vi "tower Controller.vi"(8 "error in":errorcluster) -> ()   [LabVIEW 2017]
doc: "This VI executes continuously carrying out the current operation and responding to updates or new operations. It will often contain the timing or control code that is difficult to place directly in TeleOp. This VI generally opens all sensors and motors and isolates the rest of the robot code from knowing how the operations are carried out."
uses:
  <vilib>/Rock Robotics/WPI/Framework/Completion Status.ctl
  tower Setpoints.ctl
  tower Operations.ctl
  <vilib>/Rock Robotics/SystemInterfaces/DIO/FPGA_DIOChannel.ctl
  <vilib>/Rock Robotics/WPI/Encoder/WPI_EncoderType.ctl
  <vilib>/Rock Robotics/SystemInterfaces/DIO/FPGA_DIOPWMChannel.ctl
  Phoenix-LabVIEW/Motor Controller/Controls/CTRE_Phoenix_MotorControl_ControlMode.ctl
  tower Published Globals.vi
  <vilib>/Rock Robotics/WPI/Counter/WPI_CounterDigitalInputToDigitalSource.vi
  Framework/Robot Global Data.vi
  <vilib>/Rock Robotics/WPI/PWM/WPI_PWMDeviceRef.ctl
  <vilib>/Rock Robotics/WPI/DigitalInput/WPI_DigitalInputDevRef.ctl
  <vilib>/Rock Robotics/SystemInterfaces/Encoder/FPGA_EncoderIdx.ctl
  <vilib>/Rock Robotics/SystemInterfaces/Counter/FPGA_CounterCtrSystemIndex.ctl
  <vilib>/Rock Robotics/WPI/Encoder/WPI_EncoderDevRef.ctl
  <vilib>/Rock Robotics/WPI/MotorControl/WPI_MotorControlType.ctl
  <vilib>/Rock Robotics/WPI/PWM/WPI_PWMDeadband.ctl
  <vilib>/Rock Robotics/WPI/MotorControl/WPI_MotorControlDeviceRef.ctl
  <vilib>/Rock Robotics/Network Tables/NT Write Boolean.vi
panel:
  out "Arm Encoder":dbl
  out "TowerLastCommandStatus":T1=enum."Incomplete"
  in  "Interactive Values":T2
  out "Current\nCmd":string
  in  "Buttons":cluster{"Execute Cmd":bool, "Abort Cmd":bool}
  out "Command Timing":cluster{"Start Time (ms)":u32, "Iterations":i32}
  out "Status":T1
  # "Tip: It may be helpful to observe inputs and sensor values.\nYou may also want to display tuning or debugging controls.\nFor ArmPosition Setpoint is # of raw units to travel\nFor ArmReset Setpoint is motor speed (-1 to +1)\nDuration is #seconds to run (zero is reset is immediate).\n-Motor speed sp lowers arm, + motor speed sp raises arm.\nFor reset, motor will stop when limit swtich is made."
  # "Interactive Command: You may fill in the settings for a command\nand schedule it with the Execute button. You can observe and abort\nany command while fine tuning the code for the controller."
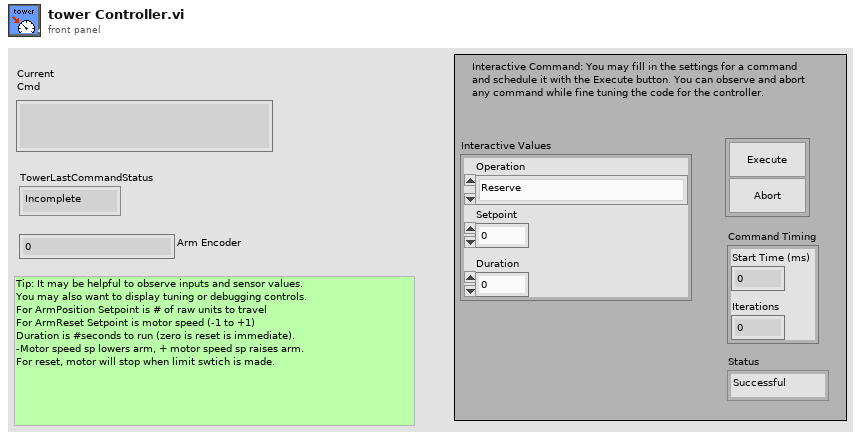
[diagram p1: front panel]
types:
  T1 = typedef "Completion Status.ctl" = enum16{"Successful", "Aborted", "Incomplete"}
  T2 = typedef "tower Setpoints.ctl" = cluster{"Operation":T3, "Setpoint":dbl, "Duration":dbl}
  T3 = typedef "tower Operations.ctl" = enum16{"Reserve", "Read Current", "Immediate", "LaunchClimber", "ArmReset", "ArmPosition", "TowerClimbImmediate", "ArmSpitPosition"}
  T4 = typedef "FPGA_DIOPWMChannel.ctl" = enum8{"PWM 0", "PWM 1", "PWM 2", "PWM 3", "PWM 4", "PWM 5", "PWM 6", "PWM 7", "PWM 8", "PWM 9", "PWM MXP 0", "PWM MXP 1", "PWM MXP 2", "PWM MXP 3", "PWM MXP 4", "PWM MXP 5", "PWM MXP 6", "PWM MXP 7", "PWM MXP 8", "PWM MXP 9", "Invalid"}
  T5 = typedef "WPI_EncoderType.ctl" = enum16{"1x", "2x", "4x"}
  T6 = typedef "FPGA_DIOChannel.ctl" = enum8{"DIO 0", "DIO 1", "DIO 2", "DIO 3", "DIO 4", "DIO 5", "DIO 6", "DIO 7", "DIO 8", "DIO 9", "DIO MXP 0", "DIO MXP 1", "DIO MXP 2", "DIO MXP 3", "DIO MXP 4", "DIO MXP 5", "DIO MXP 6", "DIO MXP 7", "DIO MXP 8", "DIO MXP 9", "DIO MXP 10", "DIO MXP 11", "DIO MXP 12", "DIO MXP 13", "DIO MXP 14", "DIO MXP 15", "SPI Port CS1", "SPI Port CS2", "SPI Port CS3", "SPI Port MISO", "SPI Port MOSI", "Invalid"}
  T7 = typedef "WPI_PWMDeviceRef.ctl" = cluster{"DeviceStatus":errorcluster, "PWM Channel":T4}
  T8 = typedef "WPI_EncoderDevRef.ctl" = cluster{"DevStatus":errorcluster, "EncoderIndex":T9, "CounterIndex":T10, "DistancePerCount":dbl, "Decoding Type":T5}
  T9 = typedef "FPGA_EncoderIdx.ctl" = enum8{"Enc 0", "Enc 1", "Enc 2", "Enc 3", "Enc 4", "Enc 5", "Enc 6", "Enc 7", "Invalid"}
  T10 = typedef "FPGA_CounterCtrSystemIndex.ctl" = enum8{"Ctr 0", "Ctr 1", "Ctr 2", "Ctr 3", "Ctr 4", "Ctr 5", "Ctr 6", "Ctr 7", "Invalid"}
  T11 = typedef "WPI_DigitalInputDevRef.ctl" = cluster{"DevStatus":errorcluster, "DIO Channel":T6}
  T12 = typedef "WPI_DigitalOutputDevRef.ctl" = cluster{"DIO Channel":T6, "DevStatus":errorcluster}
  T13 = typedef "FPGA_CounterEncoderSourceConvertionLVSourceType.ctl" = cluster{"DevStatus":errorcluster, "AnalogTriggerMode?":bool, "DigitalMode":cluster{"DIO Channel":T14}, "AnalogTriggerMode":cluster{"AnalogTriggerIndex":T15, "OutputType":T16}}
  T14 = typedef "FPGA_DIODigitalSourceChannel.ctl" = enum8{"DIO 0", "DIO 1", "DIO 2", "DIO 3", "DIO 4", "DIO 5", "DIO 6", "DIO 7", "DIO 8", "DIO 9", "DIO MXP 0", "DIO MXP 1", "DIO MXP 2", "DIO MXP 3", "DIO MXP 4", "DIO MXP 5", "DIO MXP 6", "DIO MXP 7", "DIO MXP 8", "DIO MXP 9", "DIO MXP 10", "DIO MXP 11", "DIO MXP 12", "DIO MXP 13", "DIO MXP 14", "DIO MXP 15", "Disabled"}
  T15 = typedef "FPGA_AnalogTriggerIndex.ctl" = enum8{"Trig 0", "Trig 1", "Trig 2", "Trig 3", "Trig 4", "Trig 5", "Trig 6", "Trig 7", "Invalid"}
  T16 = typedef "FPGA_AnalogTriggerOutType.ctl" = enum16{"InWindow", "TriggerState", "Rising", "Falling"}
  T17 = typedef "WPI_MotorControlDeviceRef.ctl" = cluster{"DeviceStatus":errorcluster, "Type":T18, "PWM":cluster{"PWM Channel":T4, "DeadBand":T19}, "CAN":cluster{"Device Number":u8, "SetOutput VI Ref":variant, "GetOutput VI Ref":variant, "Enable VI Ref":variant, "Disable VI Ref":variant, "Data":variant}, "Invert":bool, "DIO PWM":cluster{"PWM \"Enable\" Channel":T4, "DIOChannel":T6, "PWM Rate":dbl}}
  T18 = typedef "WPI_MotorControlType.ctl" = enum16{"PWM", "CAN", "DIO PWM"}
  T19 = typedef "WPI_PWMDeadband.ctl" = cluster{"Name":string, "maxPositivePwm":i32, "minPositivePwm":i32, "centerPwm":i32, "maxNegativePwm":i32, "minNegativePwm":i32, "angularRange":u16}
  T20 = typedef "Command Status Info.ctl" = cluster{"Name":string, "Status":T1, "notifier out":T21}
  T21 = typedef "Completion Notifier.ctl" = refnum<notifier>
  T22 = cluster{"Current Command":T2, "Command Timing":cluster{"Start Time (ms)":u32, "Iterations":i32}, "Command Arguments":cluster{"Command Info":T20, "Description":string, "Default Command":T2, "queue out":refnum<queue>, "Subsystem Name":string}}
  T23 = typedef "CTRE_Phoenix_MotorControl_ControlMode.ctl" = u16
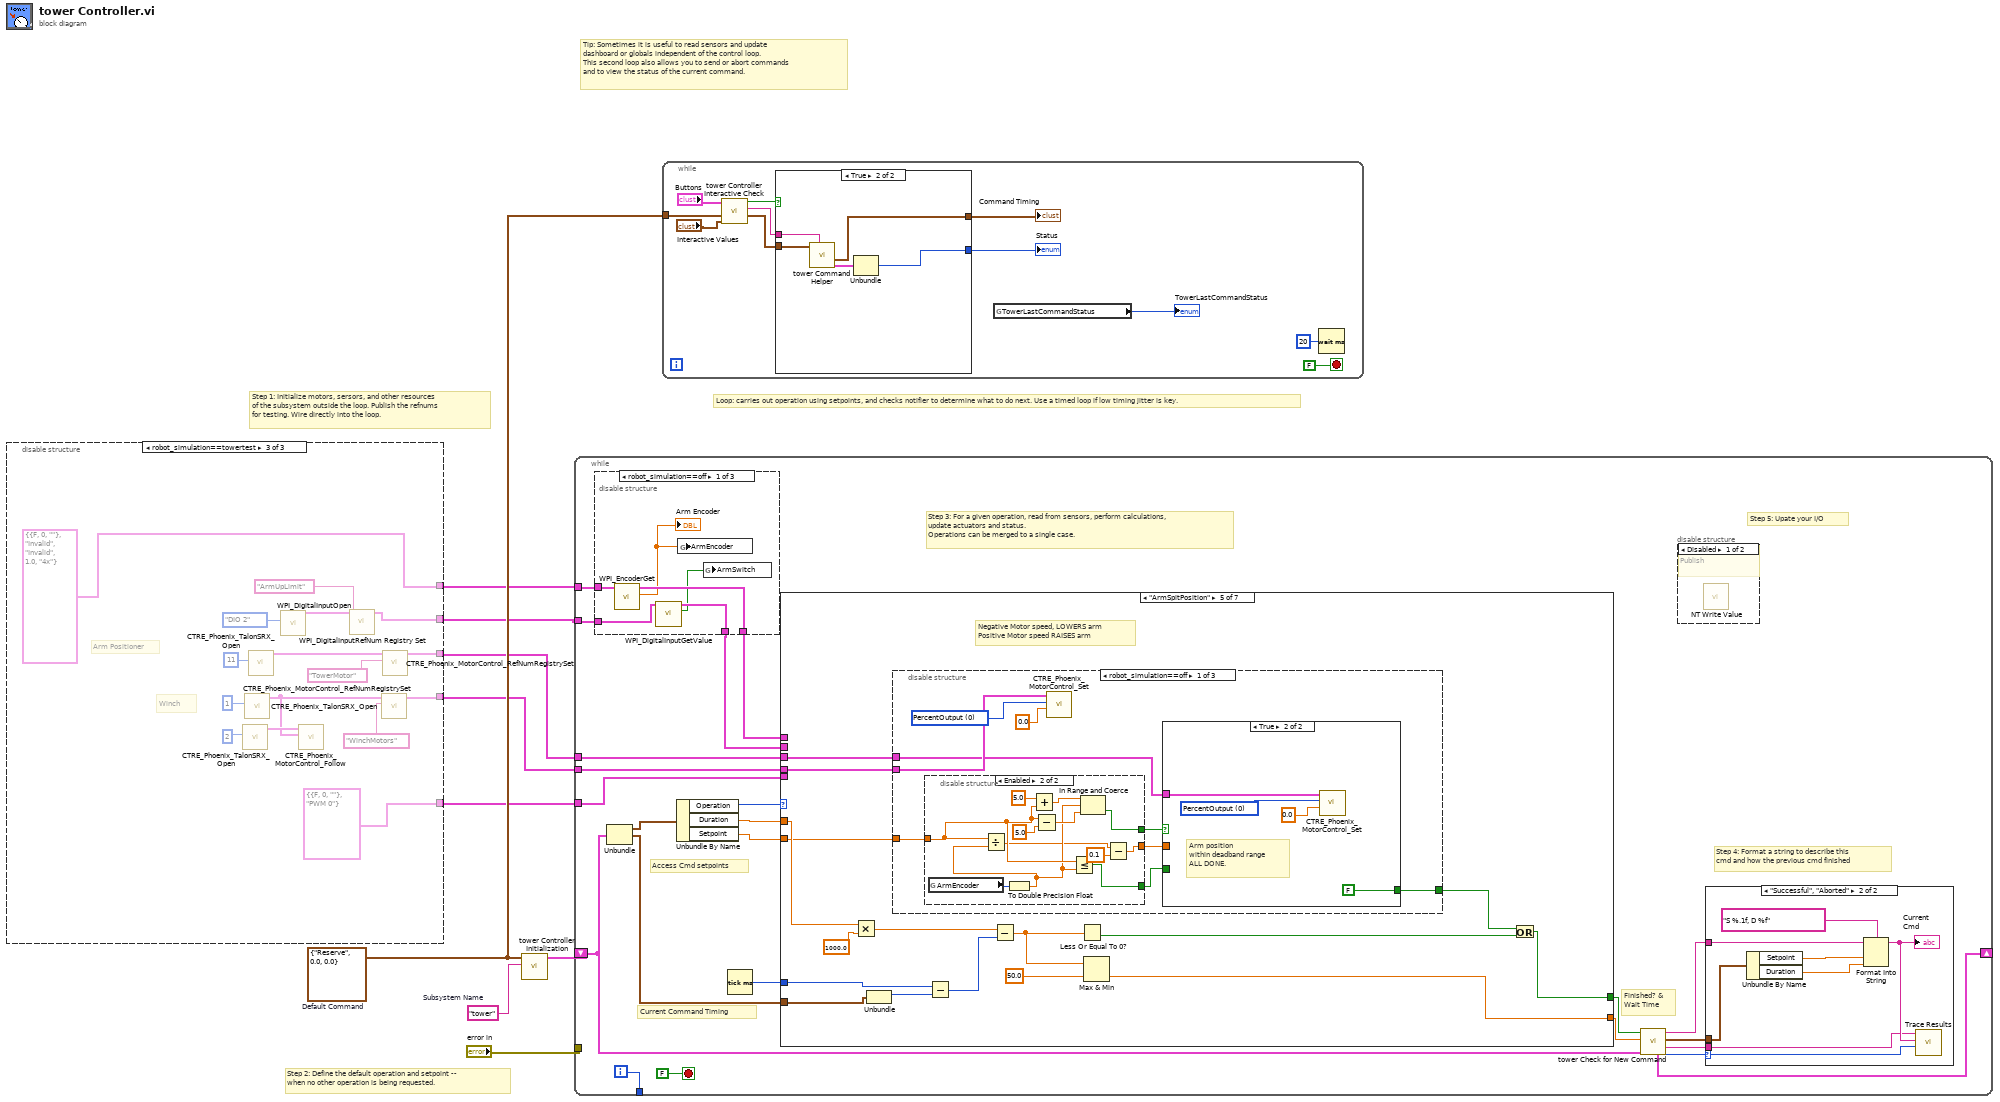
[diagram p0: block diagram]
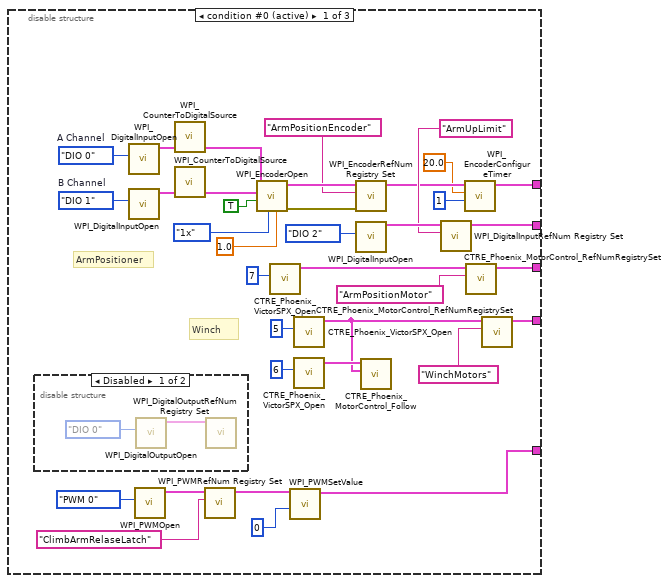
[diagram p2: hidden frame]
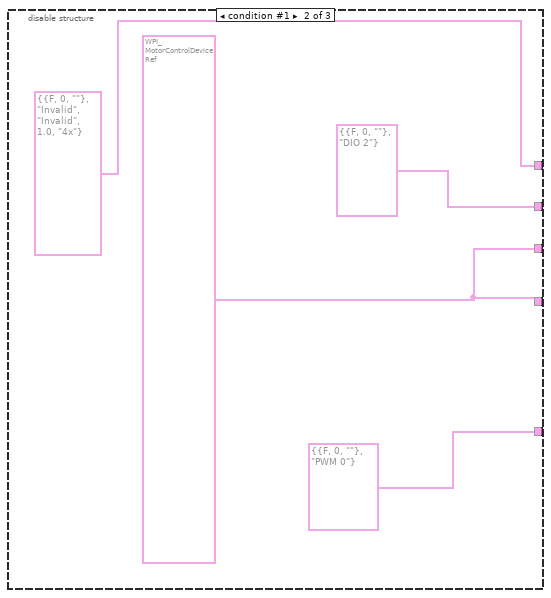
[diagram p4: hidden frame]
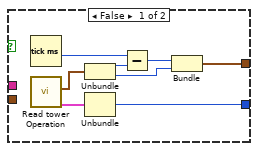
[diagram p5: hidden frame]
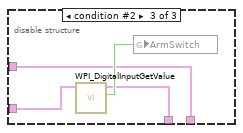
[diagram p7: hidden frame]
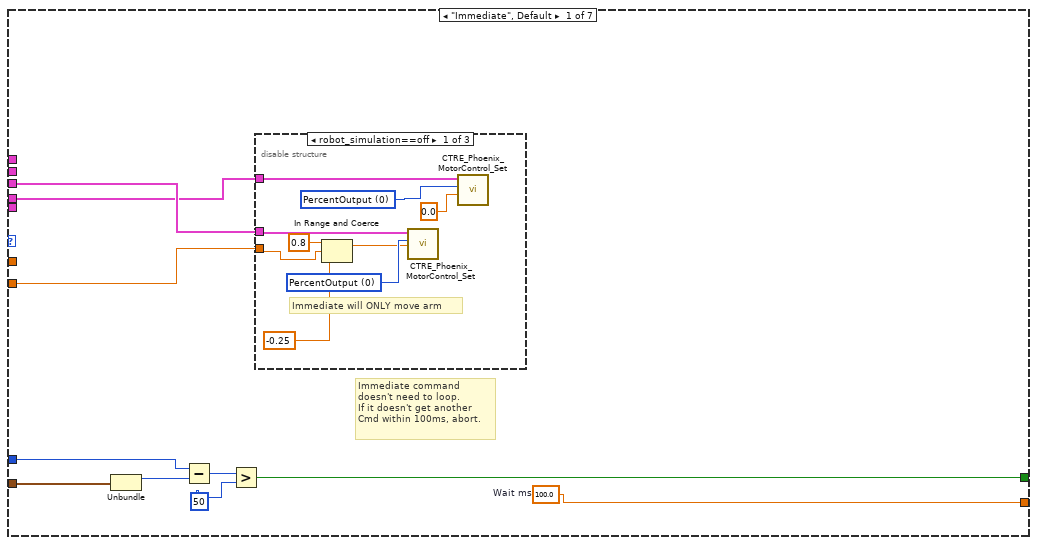
[diagram p10: hidden frame]
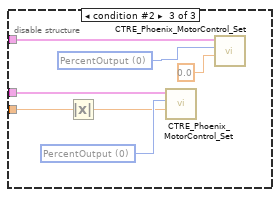
[diagram p12: hidden frame]
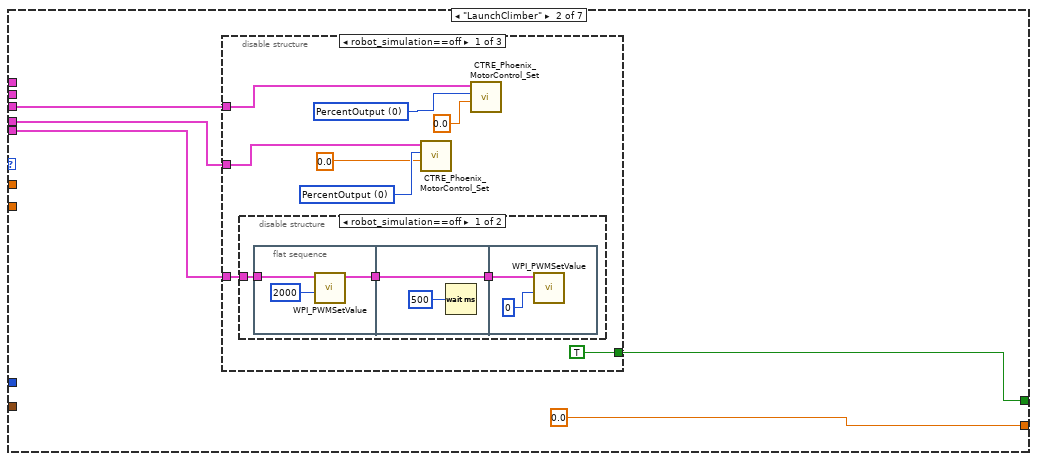
[diagram p13: hidden frame]
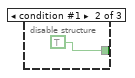
[diagram p15: hidden frame]
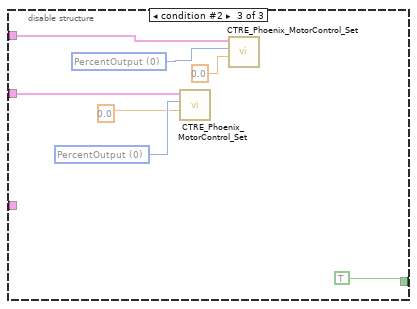
[diagram p16: hidden frame]
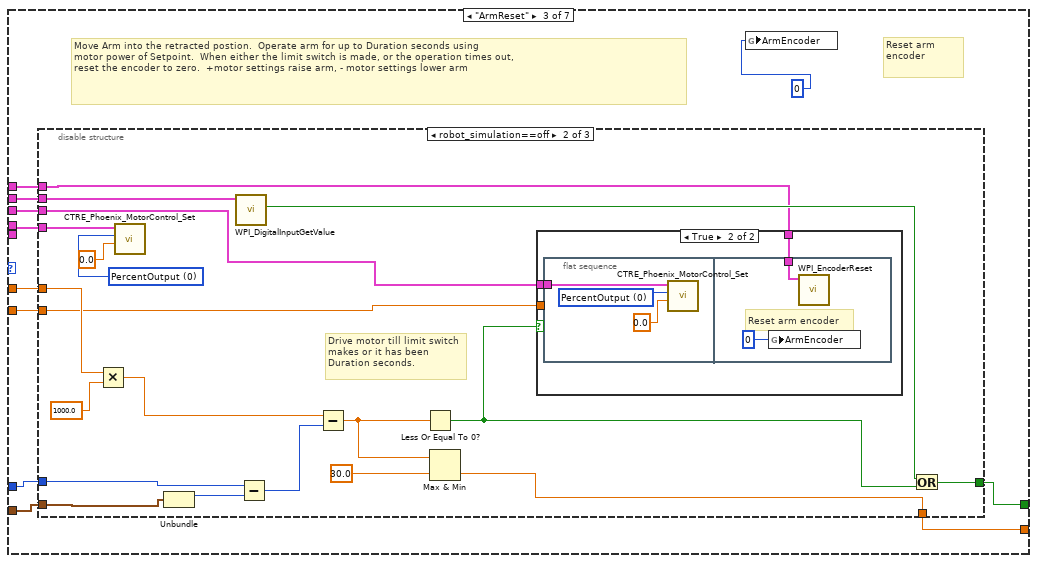
[diagram p17: hidden frame]
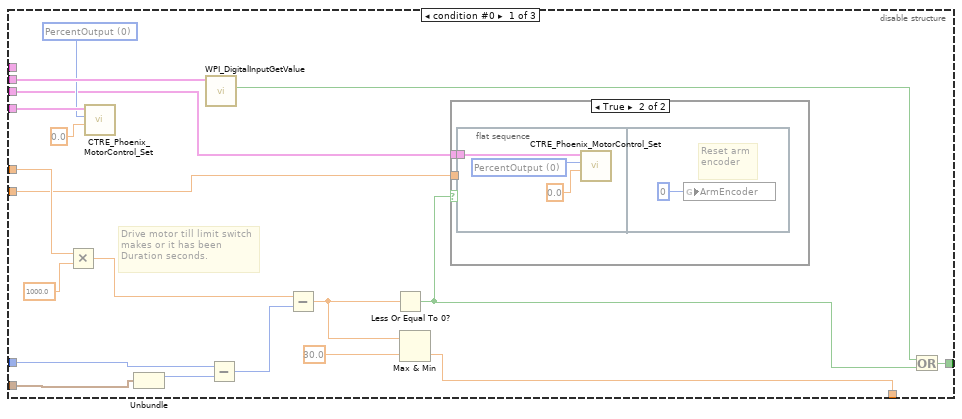
[diagram p18: hidden frame]
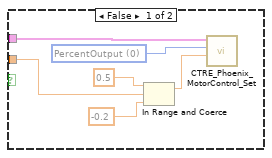
[diagram p19: hidden frame]
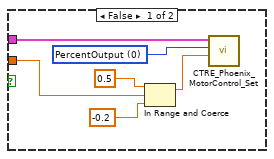
[diagram p20: hidden frame]
diagram:
  w6 = T2 {"Operation"=enum."Reserve", "Setpoint"=0.0, "Duration"=0.0}  # Default Command
  w7 = "tower"  # Subsystem Name
  # "Tip: Sometimes it is useful to read sensors and update\ndashboard or globals independent of the control loop.\nThis second loop also allows you to send or abort commands\nand to view the status of the current command."
  # "Step 2: Define the default operation and setpoint --\nwhen no other operation is being requested."
  # "Step 1: Initialize motors, sersors, and other resources\nof the subsystem outside the loop. Publish the refnums\nfor testing. Wire directly into the loop."
  # "Loop: carries out operation using setpoints, and checks notifier to determine what to do next. Use a timed loop if low timing jitter is key."
  n1 = disable-structure shown="robot_simulation==towertest" {
    disable-tunnel: [w37 w48 w65] -> w5
    disable-tunnel: [w40 w48 w61] -> w4
    disable-tunnel: [w22 T8 {"DevStatus"={"status"=FALSE, "code"=0, "source"=""}, "EncoderIndex"=enum."Invalid", "CounterIndex"=enum."Invalid", "DistancePerCount"=1.0, "Decoding Type"=enum."4x"} ("EncoderDevRef") T8 {"DevStatus"={"status"=FALSE, "code"=0, "source"=""}, "EncoderIndex"=enum."Invalid", "CounterIndex"=enum."Invalid", "DistancePerCount"=1.0, "Decoding Type"=enum."4x"} ("EncoderDevRef")] -> w1
    disable-tunnel: [w24 T11 {"DevStatus"={"status"=FALSE, "code"=0, "source"=""}, "DIO Channel"=enum."DIO 2"} ("DigitalInputDevRef") w53] -> w2
    disable-tunnel: [w13 T7 {"DeviceStatus"={"status"=FALSE, "code"=0, "source"=""}, "PWM Channel"=enum."PWM 0"} ("PWMDeviceRef") T7 {"DeviceStatus"={"status"=FALSE, "code"=0, "source"=""}, "PWM Channel"=enum."PWM 0"} ("PWMDeviceRef")] -> w3
    frame condition #0 (active) {
      w35 = FPGA_DIOChannel."DIO 1"  # B Channel
      w34 = FPGA_DIOChannel."DIO 0"  # A Channel
      # "Winch"
      # "ArmPositioner"
      n2 = disable-structure shown="Disabled" {
        frame Disabled {
          n3 = call <vilib>:"WPI_DigitalOutputOpen.vi"("DIO Channel"=FPGA_DIOChannel."DIO 0") -> ("DigitalOutputDevRef"=w47:T12)  [unwired: 9 in, 1 out]
          n4 = call <vilib>:"WPI_DigitalOutputRefNum Registry Set.vi"("DigitalOutputDevRef"=w47) -> ()  [unwired: 9 in, 2 out]
        }
        frame Enabled {
        }
      }
      n5 = call <vilib>:"WPI_DigitalInputOpen.vi"("DIO Channel"=w34) -> ("DigitalInputDevRef"=w31:T11)  [unwired: 1 in, 9 out]
      n6 = call <vilib>:"WPI_DigitalInputOpen.vi"("DIO Channel"=w35) -> ("DigitalInputDevRef"=w32:T11)  [unwired: 1 in, 9 out]
      n7 = call <vilib>:"WPI_PWMOpen.vi"("PWM Channel"=FPGA_DIOPWMChannel."PWM 0") -> ("PWMDeviceRef"=w16:T7)  [unwired: 9 in, 1 out]
      n8 = call-poly <vilib>:"WPI_CounterToDigitalSource.vi"("DigitalInputDevRef"=w31) -> ("Digital Source"=w30:T13)  [unwired: 6 out]
      n9 = call-poly <vilib>:"WPI_CounterToDigitalSource.vi"("DigitalInputDevRef"=w32) -> ("Digital Source"=w33:T13)  [unwired: 6 out]
      n10 = call <vilib>:"WPI_PWMRefNum Registry Set.vi"("refnum name"="ClimbArmRelaseLatch", "PWMDeviceRef"=w16) -> ("PWMDeviceRef"=w15:T7)  [unwired: 8 in, 1 out]
      n11 = call <vilib>:"WPI_EncoderOpen.vi"("DistancePerCount"=1.0, "Decoding Type"=WPI_EncoderType."1x", "Invert Direction (False)"=TRUE, "BSource"=w33, "ASource"=w30) -> ("error out"=w29:errorcluster, "EncoderDevRef"=w28:T8)  [unwired: 3 in, 2 out]
      n12 = call "CTRE_Phoenix_VictorSPX_Open.vi"("Device Number"=u8 7) -> ("CAN Talon SRX Ref"=w38:T17)  [unwired: 9 in, 1 out]
      n13 = call <vilib>:"WPI_PWMSetValue.vi"("Value"=u16 0, "PWMDeviceRef"=w15) -> ("PWMDeviceRef"=w13:T7)  [unwired: 8 in, 1 out]
      n14 = call "CTRE_Phoenix_VictorSPX_Open.vi"("Device Number"=u8 5) -> ("CAN Talon SRX Ref"=w41:T17)  [unwired: 9 in, 1 out]
      n15 = call "CTRE_Phoenix_VictorSPX_Open.vi"("Device Number"=u8 6) -> ("CAN Talon SRX Ref"=w42:T17)  [unwired: 9 in, 1 out]
      n16 = call <vilib>:"WPI_EncoderRefNum Registry Set.vi"("error in (no error)"=w29, "refnum name"="ArmPositionEncoder", "EncoderDevRef"=w28) -> ("EncoderDevRef"=w21:T8)  [unwired: 7 in, 1 out]
      n17 = call <vilib>:"WPI_DigitalInputOpen.vi"("DIO Channel"=FPGA_DIOChannel."DIO 2") -> ("DigitalInputDevRef"=w25:T11)  [unwired: 9 in, 1 out]
      n18 = call "CTRE_Phoenix_MotorControl_Follow.vi"("Master Controller to Follow"=w41, "PhoenixMotorControlDevRef"=w42) -> ()  [unwired: 8 in, 2 out]
      n19 = call <vilib>:"WPI_DigitalInputRefNum Registry Set.vi"("refnum name"="ArmUpLimit", "DigitalInputDevRef"=w25) -> ("DigitalInputDevRef"=w24:T11)  [unwired: 8 in, 1 out]
      n20 = call <vilib>:"WPI_EncoderConfigureTimer.vi"("Number Samples to Average"=u8 1, "Minimum Rate"=20.0, "EncoderDevRef"=w21) -> ("EncoderDevRef"=w22:T8)  [unwired: 7 in, 1 out]
      n21 = call "CTRE_Phoenix_MotorControl_RefNumRegistrySet.vi"("refnum name"="ArmPositionMotor", "PhoenixMotorControlDevRef"=w38) -> ("PhoenixMotorControlDevRef"=w37:T17)  [unwired: 8 in, 1 out]
      n22 = call "CTRE_Phoenix_MotorControl_RefNumRegistrySet.vi"("refnum name"="WinchMotors", "PhoenixMotorControlDevRef"=w41) -> ("PhoenixMotorControlDevRef"=w40:T17)  [unwired: 8 in, 1 out]
    }
    frame condition #1 {
      w48 = T17 {"DeviceStatus"={"status"=FALSE, "code"=0, "source"=""}, "Type"=enum."PWM", "PWM"={"PWM Channel"=enum."Invalid", "DeadBand"={"Name"="", "maxPositivePwm"=0, "minPositivePwm"=0, "centerPwm"=0, "maxNegativePwm"=0, "minNegativePwm"=0, "angularRange"=0}}, "CAN"={"Device Number"=0, "SetOutput VI Ref"=variant, "GetOutput VI Ref"=variant, "Enable VI Ref"=variant, "Disable VI Ref"=variant, "Data"=variant}, "Invert"=FALSE, "DIO PWM"={"PWM \"Enable\" Channel"=enum."Invalid", "DIOChannel"=enum."Invalid", "PWM Rate"=0.0}} ("PhoenixMotorControlDevRef")
    }
    frame condition #2 {
      # "Winch"
      # "Arm Positioner"
      n23 = call "CTRE_Phoenix_TalonSRX_Open.vi"("Device Number"=u8 2) -> ("CAN Talon SRX Ref"=w59:T17)  [unwired: 9 in, 1 out]
      n24 = call "CTRE_Phoenix_TalonSRX_Open.vi"("Device Number"=u8 1) -> ("CAN Talon SRX Ref"=w58:T17)  [unwired: 9 in, 1 out]
      n25 = call "CTRE_Phoenix_TalonSRX_Open.vi"("Device Number"=u8 11) -> ("CAN Talon SRX Ref"=w66:T17)  [unwired: 9 in, 1 out]
      n26 = call <vilib>:"WPI_DigitalInputOpen.vi"("DIO Channel"=FPGA_DIOChannel."DIO 2") -> ("DigitalInputDevRef"=w55:T11)  [unwired: 9 in, 1 out]
      n27 = call "CTRE_Phoenix_MotorControl_Follow.vi"("Master Controller to Follow"=w58, "PhoenixMotorControlDevRef"=w59) -> ()  [unwired: 8 in, 2 out]
      n28 = call <vilib>:"WPI_DigitalInputRefNum Registry Set.vi"("refnum name"="ArmUpLimit", "DigitalInputDevRef"=w55) -> ("DigitalInputDevRef"=w53:T11)  [unwired: 8 in, 1 out]
      n29 = call "CTRE_Phoenix_MotorControl_RefNumRegistrySet.vi"("refnum name"="WinchMotors", "PhoenixMotorControlDevRef"=w58) -> ("PhoenixMotorControlDevRef"=w61:T17)  [unwired: 8 in, 1 out]
      n30 = call "CTRE_Phoenix_MotorControl_RefNumRegistrySet.vi"("refnum name"="TowerMotor", "PhoenixMotorControlDevRef"=w66) -> ("PhoenixMotorControlDevRef"=w65:T17)  [unwired: 8 in, 1 out]
    }
  }
  n31 = call "tower Controller Initialization.vi"("Subsystem Name"=w7, "Default Command"=w6) -> ("Current Command"=w8:T22)  [unwired: 9 in]
  n32 = while {
    shift-right: [w82] -> _
    shift-left: w8 -> [w77]
    tunnel: [w89] -> _
    tunnel: "error in" -> [_]
    tunnel: w5 -> [w76]
    tunnel: w4 -> [w75]
    tunnel: w1 -> [w68]
    tunnel: w2 -> [w72]
    tunnel: w3 -> [w71]
    i -> [w89]
    stop <- FALSE stop-if-true
    # "Step 5: Upate your I/O"
    # "Step 4: Format a string to describe this\ncmd and how the previous cmd finished"
    # "Current Command Timing"
    # "Access Cmd setpoints"
    # "Finished? &\nWait Time"
    # "Step 3: For a given operation, read from sensors, perform calculations,\nupdate actuators and status.\nOperations can be merged to a single case."
    n33 = disable-structure shown="robot_simulation==off" {
      disable-tunnel: w68 -> [w92 w98 w99]
      disable-tunnel: [w96 w98 w99] -> w74
      disable-tunnel: w72 -> [w95 w97 w101]
      disable-tunnel: [w94 w97 w100] -> w73
      frame condition #0 (active) {
        n34 = call <vilib>:"WPI_EncoderGet.vi"("EncoderDevRef"=w92) -> ("Distance"=w91:dbl, "EncoderDevRef"=w96:T8)  [unwired: 5 in, 4 out]
        "Arm Encoder" <- w91
        n35 = call <vilib>:"WPI_DigitalInputGetValue.vi"("DigitalInputDevRef"=w95) -> ("Value"=w93:bool, "DigitalInputDevRef"=w94:T11)  [unwired: 8 in, 1 out]
        n36 = global write "Robot Global Data.vi" "ArmEncoder"(w91) -> ()
        n37 = global write "Robot Global Data.vi" "ArmSwitch"(w93) -> ()
      }
      frame condition #1 {
      }
      frame condition #2 {
        n38 = call <vilib>:"WPI_DigitalInputGetValue.vi"("DigitalInputDevRef"=w101) -> ("Value"=w102:bool, "DigitalInputDevRef"=w100:T11)  [unwired: 8 in, 1 out]
        n39 = global write "Robot Global Data.vi" "ArmSwitch"(w102) -> ()
      }
    }
    n40 = Unbundle(w77) -> ("Current Command"=w88:T2, "Command Timing"=w84:cluster{"Start Time (ms)":u32, "Iterations":i32})  [unwired: 1 out]
    n41 = Unbundle By Name(w88) -> ("Operation"=w87:T3, "Duration"=w86:dbl, "Setpoint"=w83:dbl)
    n42 = Tick Count (ms)() -> (millisecond timer value=w85:u32)
    n43 = case shown="\"ArmSpitPosition\"" w87 {
      tunnel: [w120 0.0 ("Infinite") w169 w253 w301 100.0 w379] -> w69
      tunnel: [w114 w137 w170 w250 w298 FALSE ("ignore previous (F)") w380] -> w70
      tunnel: w84 -> [w116 _ w172 w255 w303 _ w382]
      tunnel: w86 -> [_ _ w174 w252 w300 _ _]
      tunnel: w85 -> [w115 _ w171 w254 w302 _ w381]
      tunnel: w83 -> [w112 _ w173 w247 w295 _ w378]
      tunnel: w76 -> [w113 w139 w177 w246 w294 w363 w376]
      tunnel: w75 -> [w111 w140 w175 w251 w299 w362 w377]
      tunnel: w74 -> [_ _ w176 _ _ _ _]
      tunnel: w73 -> [_ _ w178 _ _ _ _]
      tunnel: w71 -> [_ w138 _ _ _ _ _]
      frame "Immediate", Default {
        w120 = 100.0  # Wait ms
        # "Immediate command\ndoesn't need to loop.\nIf it doesn't get another\nCmd within 100ms, abort."
        n44 = Unbundle(w116) -> ("Start Time (ms)"=w119:u32)  [unwired: 1 out]
        n45 = Subtract(x=w115, y=w119) -> (x-y=w118:u32)
        n46 = Greater?(x=w118, y=u8 50 ("Left Motor")) -> (0:w114:bool)
        n47 = disable-structure shown="robot_simulation==off" {
          disable-tunnel: w113 -> [w129 _ w136]
          disable-tunnel: w112 -> [w122 _ w134]
          disable-tunnel: w111 -> [w125 _ w130]
          frame condition #0 (active) {
            w126 = T23 0 items=["PercentOutput"=0, "Position"=1, "Velocity"=2, "Current"=3, "Follower"=5, "MotionProfile"=6, "MotionMagic"=7, "MotionMagicArc"=8, "MotionProfileArc"=10, "Disabled"=15] ("Control Mode")
            w128 = T23 0 items=["PercentOutput"=0, "Position"=1, "Velocity"=2, "Current"=3, "Follower"=5, "MotionProfile"=6, "MotionMagic"=7, "MotionMagicArc"=8, "MotionProfileArc"=10, "Disabled"=15] ("Control Mode")
            # "Immediate will ONLY move arm"
            n48 = In Range and Coerce(upper limit=0.8, x=w122, lower limit=-0.25) -> (coerced(x)=w121:dbl)  [unwired: 1 out]
            n49 = call "CTRE_Phoenix_MotorControl_Set.vi"("Output"=w121, "Control Mode"=w128, "PhoenixMotorControlDevRef"=w129) -> ()  [unwired: 7 in, 2 out]
            n50 = call "CTRE_Phoenix_MotorControl_Set.vi"("Output"=0.0, "Control Mode"=w126, "PhoenixMotorControlDevRef"=w125) -> ()  [unwired: 7 in, 2 out]
          }
          frame condition #1 {
          }
          frame condition #2 {
            w131 = T23 0 items=["PercentOutput"=0, "Position"=1, "Velocity"=2, "Current"=3, "Follower"=5, "MotionProfile"=6, "MotionMagic"=7, "MotionMagicArc"=8, "MotionProfileArc"=10, "Disabled"=15] ("Control Mode")
            w135 = T23 0 items=["PercentOutput"=0, "Position"=1, "Velocity"=2, "Current"=3, "Follower"=5, "MotionProfile"=6, "MotionMagic"=7, "MotionMagicArc"=8, "MotionProfileArc"=10, "Disabled"=15] ("Control Mode")
            n51 = Absolute Value(x=w134) -> (abs(x)=w133:dbl)
            n52 = call "CTRE_Phoenix_MotorControl_Set.vi"("Output"=w133, "Control Mode"=w135, "PhoenixMotorControlDevRef"=w136) -> ()  [unwired: 7 in, 2 out]
            n53 = call "CTRE_Phoenix_MotorControl_Set.vi"("Output"=0.0, "Control Mode"=w131, "PhoenixMotorControlDevRef"=w130) -> ()  [unwired: 7 in, 2 out]
          }
        }
      }
      frame "LaunchClimber" {
        n54 = disable-structure shown="robot_simulation==off" {
          disable-tunnel: w140 -> [w144 _ w167]
          disable-tunnel: w139 -> [w145 _ w163]
          disable-tunnel: w138 -> [w143 _ _]
          disable-tunnel: [TRUE ("ignore previous (F)") TRUE ("ignore previous (F)") TRUE ("ignore previous (F)")] -> w137
          frame condition #0 (active) {
            w147 = T23 0 items=["PercentOutput"=0, "Position"=1, "Velocity"=2, "Current"=3, "Follower"=5, "MotionProfile"=6, "MotionMagic"=7, "MotionMagicArc"=8, "MotionProfileArc"=10, "Disabled"=15] ("Control Mode")
            w149 = T23 0 items=["PercentOutput"=0, "Position"=1, "Velocity"=2, "Current"=3, "Follower"=5, "MotionProfile"=6, "MotionMagic"=7, "MotionMagicArc"=8, "MotionProfileArc"=10, "Disabled"=15] ("Control Mode")
            n55 = disable-structure shown="robot_simulation==off" {
              disable-tunnel: w143 -> [w150 _]
              frame condition #0 (active) {
                n56 = flat-sequence {
                  tunnel: w150 -> [w154]
                  tunnel: [w155] -> w152
                  tunnel: [w156] -> w151
                  tunnel: w152 -> [w156]
                  tunnel: w151 -> [w159]
                  frame #0 {
                    n57 = call <vilib>:"WPI_PWMSetValue.vi"("Value"=u16 2000, "PWMDeviceRef"=w154) -> ("PWMDeviceRef"=w155:T7)  [unwired: 8 in, 1 out]
                  }
                  frame #1 {
                    n58 = Wait (ms)(milliseconds to wait=u32 500) -> ()  [unwired: 1 out]
                  }
                  frame #2 {
                    n59 = call <vilib>:"WPI_PWMSetValue.vi"("Value"=u16 0, "PWMDeviceRef"=w159) -> ()  [unwired: 8 in, 2 out]
                  }
                }
              }
              frame condition #1 {
              }
            }
            n60 = call "CTRE_Phoenix_MotorControl_Set.vi"("Output"=0.0, "Control Mode"=w149, "PhoenixMotorControlDevRef"=w144) -> ()  [unwired: 7 in, 2 out]
            n61 = call "CTRE_Phoenix_MotorControl_Set.vi"("Output"=0.0, "Control Mode"=w147, "PhoenixMotorControlDevRef"=w145) -> ()  [unwired: 7 in, 2 out]
          }
          frame condition #1 {
          }
          frame condition #2 {
            w164 = T23 0 items=["PercentOutput"=0, "Position"=1, "Velocity"=2, "Current"=3, "Follower"=5, "MotionProfile"=6, "MotionMagic"=7, "MotionMagicArc"=8, "MotionProfileArc"=10, "Disabled"=15] ("Control Mode")
            w166 = T23 0 items=["PercentOutput"=0, "Position"=1, "Velocity"=2, "Current"=3, "Follower"=5, "MotionProfile"=6, "MotionMagic"=7, "MotionMagicArc"=8, "MotionProfileArc"=10, "Disabled"=15] ("Control Mode")
            n62 = call "CTRE_Phoenix_MotorControl_Set.vi"("Output"=0.0, "Control Mode"=w166, "PhoenixMotorControlDevRef"=w167) -> ()  [unwired: 7 in, 2 out]
            n63 = call "CTRE_Phoenix_MotorControl_Set.vi"("Output"=0.0, "Control Mode"=w164, "PhoenixMotorControlDevRef"=w163) -> ()  [unwired: 7 in, 2 out]
          }
        }
      }
      frame "ArmReset" {
        # "Reset arm \nencoder"
        # "Move Arm into the retracted postion.  Operate arm for up to Duration seconds using\nmotor power of Setpoint.  When either the limit switch is made, or the operation times out,\nreset the encoder to zero.  +motor settings raise arm, - motor settings lower arm"
        n64 = disable-structure shown="robot_simulation==off" {
          disable-tunnel: w178 -> [w197 w228 _]
          disable-tunnel: w177 -> [w180 w211 _]
          disable-tunnel: w176 -> [_ w209 _]
          disable-tunnel: w175 -> [w196 w227 _]
          disable-tunnel: w174 -> [w183 w214 _]
          disable-tunnel: w173 -> [w179 w210 _]
          disable-tunnel: w172 -> [w189 w220 _]
          disable-tunnel: w171 -> [w188 w219 _]
          disable-tunnel: [w186 w217 TRUE] -> w170
          disable-tunnel: [w185 w216 -1.0] -> w169
          frame condition #0 {
            w194 = T23 0 items=["PercentOutput"=0, "Position"=1, "Velocity"=2, "Current"=3, "Follower"=5, "MotionProfile"=6, "MotionMagic"=7, "MotionMagicArc"=8, "MotionProfileArc"=10, "Disabled"=15] ("Control Mode")
            # "Drive motor till limit switch makes or it has been Duration seconds."
            n65 = Multiply(x=w183, y=1000.0) -> (x*y=w182:dbl)
            n66 = call "CTRE_Phoenix_MotorControl_Set.vi"("Output"=0.0, "Control Mode"=w194, "PhoenixMotorControlDevRef"=w196) -> ()  [unwired: 7 in, 2 out]
            n67 = Unbundle(w189) -> ("Start Time (ms)"=w192:u32)  [unwired: 1 out]
            n68 = call <vilib>:"WPI_DigitalInputGetValue.vi"("DigitalInputDevRef"=w197) -> ("Value"=w187:bool)  [unwired: 8 in, 2 out]
            n69 = Subtract(x=w188, y=w192) -> (x-y=w193:u32)
            n70 = Subtract(x=w182, y=w193) -> (x-y=w191:dbl)
            n71 = Less Or Equal To 0?(x=w191) -> (x <= 0?=w181:bool)
            n72 = Max & Min(x=w191, y=30.0) -> (min(x,y)=w185:dbl)  [unwired: 1 out]
            n73 = case shown="True" w181 {
              tunnel: w180 -> [w199 w204]
              tunnel: w179 -> [w198 _]
              frame False {
                w203 = T23 0 items=["PercentOutput"=0, "Position"=1, "Velocity"=2, "Current"=3, "Follower"=5, "MotionProfile"=6, "MotionMagic"=7, "MotionMagicArc"=8, "MotionProfileArc"=10, "Disabled"=15] ("Control Mode")
                n74 = In Range and Coerce(upper limit=0.5, x=w198, lower limit=-0.2) -> (coerced(x)=w202:dbl)  [unwired: 1 out]
                n75 = call "CTRE_Phoenix_MotorControl_Set.vi"("Output"=w202, "Control Mode"=w203, "PhoenixMotorControlDevRef"=w199) -> ()  [unwired: 7 in, 2 out]
              }
              frame True {
                n76 = flat-sequence {
                  tunnel: w204 -> [w205]
                  frame #0 {
                    w207 = T23 0 items=["PercentOutput"=0, "Position"=1, "Velocity"=2, "Current"=3, "Follower"=5, "MotionProfile"=6, "MotionMagic"=7, "MotionMagicArc"=8, "MotionProfileArc"=10, "Disabled"=15] ("Control Mode")
                    n77 = call "CTRE_Phoenix_MotorControl_Set.vi"("Output"=0.0, "Control Mode"=w207, "PhoenixMotorControlDevRef"=w205) -> ()  [unwired: 7 in, 2 out]
                  }
                  frame #1 {
                    # "Reset arm \nencoder"
                    n78 = global write "Robot Global Data.vi" "ArmEncoder"(0 ("ArmEncoder")) -> ()
                  }
                }
              }
            }
            n79 = Or(x=w187, y=w181) -> (x .or. y?=w186:bool)
          }
          frame condition #1 (active) {
            w225 = T23 0 items=["PercentOutput"=0, "Position"=1, "Velocity"=2, "Current"=3, "Follower"=5, "MotionProfile"=6, "MotionMagic"=7, "MotionMagicArc"=8, "MotionProfileArc"=10, "Disabled"=15] ("Control Mode")
            # "Drive motor till limit switch makes or it has been Duration seconds."
            n80 = Multiply(x=w214, y=1000.0) -> (x*y=w213:dbl)
            n81 = call "CTRE_Phoenix_MotorControl_Set.vi"("Output"=0.0, "Control Mode"=w225, "PhoenixMotorControlDevRef"=w227) -> ()  [unwired: 7 in, 2 out]
            n82 = Unbundle(w220) -> ("Start Time (ms)"=w223:u32)  [unwired: 1 out]
            n83 = call <vilib>:"WPI_DigitalInputGetValue.vi"("DigitalInputDevRef"=w228) -> ("Value"=w218:bool)  [unwired: 8 in, 2 out]
            n84 = Subtract(x=w219, y=w223) -> (x-y=w224:u32)
            n85 = Subtract(x=w213, y=w224) -> (x-y=w222:dbl)
            n86 = Less Or Equal To 0?(x=w222) -> (x <= 0?=w212:bool)
            n87 = Max & Min(x=w222, y=30.0) -> (min(x,y)=w216:dbl)  [unwired: 1 out]
            n88 = case shown="True" w212 {
              tunnel: w211 -> [w230 w236]
              tunnel: w210 -> [w229 _]
              tunnel: w209 -> [_ w235]
              frame False {
                w234 = T23 0 items=["PercentOutput"=0, "Position"=1, "Velocity"=2, "Current"=3, "Follower"=5, "MotionProfile"=6, "MotionMagic"=7, "MotionMagicArc"=8, "MotionProfileArc"=10, "Disabled"=15] ("Control Mode")
                n89 = In Range and Coerce(upper limit=0.5, x=w229, lower limit=-0.2) -> (coerced(x)=w233:dbl)  [unwired: 1 out]
                n90 = call "CTRE_Phoenix_MotorControl_Set.vi"("Output"=w233, "Control Mode"=w234, "PhoenixMotorControlDevRef"=w230) -> ()  [unwired: 7 in, 2 out]
              }
              frame True {
                n91 = flat-sequence {
                  tunnel: w236 -> [w237]
                  tunnel: w235 -> [w240]
                  frame #0 {
                    w239 = T23 0 items=["PercentOutput"=0, "Position"=1, "Velocity"=2, "Current"=3, "Follower"=5, "MotionProfile"=6, "MotionMagic"=7, "MotionMagicArc"=8, "MotionProfileArc"=10, "Disabled"=15] ("Control Mode")
                    n92 = call "CTRE_Phoenix_MotorControl_Set.vi"("Output"=0.0, "Control Mode"=w239, "PhoenixMotorControlDevRef"=w237) -> ()  [unwired: 7 in, 2 out]
                  }
                  frame #1 {
                    # "Reset arm encoder"
                    n93 = global write "Robot Global Data.vi" "ArmEncoder"(0 ("ArmEncoder")) -> ()
                    n94 = call <vilib>:"WPI_EncoderReset.vi"("EncoderDevRef"=w240) -> ()  [unwired: 9 in, 2 out]
                  }
                }
              }
            }
            n95 = Or(x=w218, y=w212) -> (x .or. y?=w217:bool)
          }
          frame condition #2 {
            n96 = global write "Robot Global Data.vi" "ArmEncoder"(0 ("ArmEncoder")) -> ()
          }
        }
        n97 = global write "Robot Global Data.vi" "ArmEncoder"(0 ("ArmEncoder")) -> ()
      }
      frame "ArmPosition" {
        # "Negative Motor speed, LOWERS arm\nPositive Motor speed RAISES arm"
        n98 = disable-structure shown="robot_simulation==off" {
          disable-tunnel: w251 -> [w275 w288 _]
          disable-tunnel: [w268 _ _] -> w248
          disable-tunnel: w247 -> [w267 _ _]
          disable-tunnel: w246 -> [w263 w287 _]
          frame condition #0 (active) {
            w261 = T23 0 items=["PercentOutput"=0, "Position"=1, "Velocity"=2, "Current"=3, "Follower"=5, "MotionProfile"=6, "MotionMagic"=7, "MotionMagicArc"=8, "MotionProfileArc"=10, "Disabled"=15] ("Control Mode")
            n99 = global read "Robot Global Data.vi" "ArmEncoder"() -> (w270:i32)
            n100 = Add(x=5.0, y=w267) -> (x+y=w274:dbl)
            n101 = Subtract(x=w267, y=5.0 ("x")) -> (x-y=w271:dbl)
            n102 = To Double Precision Float(number=w270) -> (double precision float=w266:dbl)
            n103 = Subtract(x=w267, y=w266) -> (x-y=w265:dbl)
            n104 = In Range and Coerce(upper limit=w274, x=w266, lower limit=w271) -> (In Range?=w269:bool)  [unwired: 1 out]
            n105 = Less Than 0?(x=w265) -> (x < 0?=w264:bool)
            n106 = case shown="False" w269 {
              tunnel: [FALSE TRUE] -> w268
              tunnel: w264 -> [w278 _]
              tunnel: w263 -> [w276 w285]
              frame False {
                w279 = T23 0 items=["PercentOutput"=0, "Position"=1, "Velocity"=2, "Current"=3, "Follower"=5, "MotionProfile"=6, "MotionMagic"=7, "MotionMagicArc"=8, "MotionProfileArc"=10, "Disabled"=15] ("Control Mode")
                # "Not in range, keep moving"
                n107 = case shown="False" w278 {
                  tunnel: [-0.25 ("Output") 0.8 ("Output")] -> w277
                  frame False {
                    # "lower more"
                  }
                  frame True {
                    # "raise more"
                  }
                }
                n108 = call "CTRE_Phoenix_MotorControl_Set.vi"("Output"=w277, "Control Mode"=w279, "PhoenixMotorControlDevRef"=w276) -> ()  [unwired: 7 in, 2 out]
              }
              frame True {
                w284 = T23 0 items=["PercentOutput"=0, "Position"=1, "Velocity"=2, "Current"=3, "Follower"=5, "MotionProfile"=6, "MotionMagic"=7, "MotionMagicArc"=8, "MotionProfileArc"=10, "Disabled"=15] ("Control Mode")
                # "Arm position\nwithin deadband range\nALL DONE."
                n109 = call "CTRE_Phoenix_MotorControl_Set.vi"("Output"=0.0, "Control Mode"=w284, "PhoenixMotorControlDevRef"=w285) -> ()  [unwired: 7 in, 2 out]
              }
            }
            n110 = call "CTRE_Phoenix_MotorControl_Set.vi"("Output"=0.0, "Control Mode"=w261, "PhoenixMotorControlDevRef"=w275) -> ()  [unwired: 7 in, 2 out]
          }
          frame condition #1 {
            w290 = T23 0 items=["PercentOutput"=0, "Position"=1, "Velocity"=2, "Current"=3, "Follower"=5, "MotionProfile"=6, "MotionMagic"=7, "MotionMagicArc"=8, "MotionProfileArc"=10, "Disabled"=15] ("Control Mode")
            w291 = T23 0 items=["PercentOutput"=0, "Position"=1, "Velocity"=2, "Current"=3, "Follower"=5, "MotionProfile"=6, "MotionMagic"=7, "MotionMagicArc"=8, "MotionProfileArc"=10, "Disabled"=15] ("Control Mode")
            n111 = call "CTRE_Phoenix_MotorControl_Set.vi"("Output"=0.0, "Control Mode"=w291, "PhoenixMotorControlDevRef"=w288) -> ()  [unwired: 7 in, 2 out]
            n112 = call "CTRE_Phoenix_MotorControl_Set.vi"("Output"=0.0, "Control Mode"=w290, "PhoenixMotorControlDevRef"=w287) -> ()  [unwired: 7 in, 2 out]
          }
          frame condition #2 {
          }
        }
        n113 = Multiply(x=w252, y=1000.0) -> (x*y=w259:dbl)
        n114 = Unbundle(w255) -> ("Start Time (ms)"=w258:u32)  [unwired: 1 out]
        n115 = Subtract(x=w254, y=w258) -> (x-y=w260:u32)
        n116 = Subtract(x=w259, y=w260) -> (x-y=w257:dbl)
        n117 = Less Or Equal To 0?(x=w257) -> (x <= 0?=w249:bool)
        n118 = Max & Min(x=w257, y=50.0) -> (min(x,y)=w253:dbl)  [unwired: 1 out]
        n119 = Or(x=w248, y=w249) -> (x .or. y?=w250:bool)
      }
      frame "ArmSpitPosition" {
        # "Negative Motor speed, LOWERS arm\nPositive Motor speed RAISES arm"
        n120 = Multiply(x=w300, y=1000.0) -> (x*y=w307:dbl)
        n121 = Unbundle(w303) -> ("Start Time (ms)"=w306:u32)  [unwired: 1 out]
        n122 = disable-structure shown="robot_simulation==off" {
          disable-tunnel: w299 -> [w317 w356 _]
          disable-tunnel: [w315 _ _] -> w296
          disable-tunnel: w295 -> [w314 _ _]
          disable-tunnel: w294 -> [w312 w355 _]
          frame condition #0 (active) {
            w310 = T23 0 items=["PercentOutput"=0, "Position"=1, "Velocity"=2, "Current"=3, "Follower"=5, "MotionProfile"=6, "MotionMagic"=7, "MotionMagicArc"=8, "MotionProfileArc"=10, "Disabled"=15] ("Control Mode")
            n123 = disable-structure shown="Enabled" {
              disable-tunnel: [w322 w333] -> w316
              disable-tunnel: w314 -> [w321 w335]
              disable-tunnel: [w318 w338] -> w313
              disable-tunnel: [_ w328] -> w309
              frame Disabled {
                n124 = global read "Robot Global Data.vi" "ArmEncoder"() -> (w323:i32)
                n125 = Add(x=5.0, y=w321) -> (x+y=w327:dbl)
                n126 = Subtract(x=w321, y=5.0 ("x")) -> (x-y=w324:dbl)
                n127 = To Double Precision Float(number=w323) -> (double precision float=w320:dbl)
                n128 = Subtract(x=w321, y=w320) -> (x-y=w319:dbl)
                n129 = In Range and Coerce(upper limit=w327, x=w320, lower limit=w324) -> (In Range?=w322:bool)  [unwired: 1 out]
                n130 = Less Than 0?(x=w319) -> (x < 0?=w318:bool)
              }
              frame Enabled {
                n131 = global read "Robot Global Data.vi" "ArmEncoder"() -> (w339:i32)
                n132 = To Double Precision Float(number=w339) -> (double precision float=w331:dbl)
                n133 = Divide(x=w335, y=w331) -> (x/y=w330:dbl)
                n134 = Add(x=5.0, y=w335) -> (x+y=w336:dbl)
                n135 = Subtract(x=w335, y=5.0) -> (x-y=w332:dbl)
                n136 = Less Or Equal?(x=w335, y=w331) -> (x <= y?=w338:bool)
                n137 = In Range and Coerce(upper limit=w336, x=w331, lower limit=w332) -> (In Range?=w333:bool)  [unwired: 1 out]
                n138 = Subtract(x=w330, y=0.1) -> (x-y=w328:dbl)
              }
            }
            n139 = call "CTRE_Phoenix_MotorControl_Set.vi"("Output"=0.0, "Control Mode"=w310, "PhoenixMotorControlDevRef"=w317) -> ()  [unwired: 7 in, 2 out]
            n140 = case shown="True" w316 {
              tunnel: [FALSE FALSE] -> w315
              tunnel: w313 -> [w343 _]
              tunnel: w312 -> [w341 w353]
              tunnel: w309 -> [w340 _]
              frame False {
                w344 = T23 0 items=["PercentOutput"=0, "Position"=1, "Velocity"=2, "Current"=3, "Follower"=5, "MotionProfile"=6, "MotionMagic"=7, "MotionMagicArc"=8, "MotionProfileArc"=10, "Disabled"=15] ("Control Mode")
                # "Not in range, keep moving"
                n141 = case shown="True" w343 {
                  tunnel: [-0.1 ("Output") w350] -> w342
                  tunnel: w340 -> [_ w347]
                  frame False {
                    # "lower more"
                  }
                  frame True {
                    # "raise more"
                    n142 = In Range and Coerce(upper limit=0.7, x=w347, lower limit=0.0) -> (coerced(x)=w350:dbl)  [unwired: 1 out]
                  }
                }
                n143 = call "CTRE_Phoenix_MotorControl_Set.vi"("Output"=w342, "Control Mode"=w344, "PhoenixMotorControlDevRef"=w341) -> ()  [unwired: 7 in, 2 out]
              }
              frame True {
                w352 = T23 0 items=["PercentOutput"=0, "Position"=1, "Velocity"=2, "Current"=3, "Follower"=5, "MotionProfile"=6, "MotionMagic"=7, "MotionMagicArc"=8, "MotionProfileArc"=10, "Disabled"=15] ("Control Mode")
                # "Arm position\nwithin deadband range\nALL DONE."
                n144 = call "CTRE_Phoenix_MotorControl_Set.vi"("Output"=0.0, "Control Mode"=w352, "PhoenixMotorControlDevRef"=w353) -> ()  [unwired: 7 in, 2 out]
              }
            }
          }
          frame condition #1 {
            w358 = T23 0 items=["PercentOutput"=0, "Position"=1, "Velocity"=2, "Current"=3, "Follower"=5, "MotionProfile"=6, "MotionMagic"=7, "MotionMagicArc"=8, "MotionProfileArc"=10, "Disabled"=15] ("Control Mode")
            w359 = T23 0 items=["PercentOutput"=0, "Position"=1, "Velocity"=2, "Current"=3, "Follower"=5, "MotionProfile"=6, "MotionMagic"=7, "MotionMagicArc"=8, "MotionProfileArc"=10, "Disabled"=15] ("Control Mode")
            n145 = call "CTRE_Phoenix_MotorControl_Set.vi"("Output"=0.0, "Control Mode"=w359, "PhoenixMotorControlDevRef"=w356) -> ()  [unwired: 7 in, 2 out]
            n146 = call "CTRE_Phoenix_MotorControl_Set.vi"("Output"=0.0, "Control Mode"=w358, "PhoenixMotorControlDevRef"=w355) -> ()  [unwired: 7 in, 2 out]
          }
          frame condition #2 {
          }
        }
        n147 = Subtract(x=w302, y=w306) -> (x-y=w308:u32)
        n148 = Subtract(x=w307, y=w308) -> (x-y=w305:dbl)
        n149 = Less Or Equal To 0?(x=w305) -> (x <= 0?=w297:bool)
        n150 = Max & Min(x=w305, y=50.0) -> (min(x,y)=w301:dbl)  [unwired: 1 out]
        n151 = Or(x=w296, y=w297) -> (x .or. y?=w298:bool)
      }
      frame "Reserve" {
        # "Encoder needs to be polled,\nuse 100ms wait for command\nbefore checking sensors"
        # "If loop needs to poll sensors or other\nvalues, use a timeout value. -1 waits for\nnext command to be sent."
        n152 = disable-structure shown="robot_simulation==towertest" {
          disable-tunnel: w363 -> [w369 _ w374]
          disable-tunnel: w362 -> [w368 _ w372]
          disable-tunnel: 0.0 ("Output") -> [w366 _ w371]
          frame condition #0 (active) {
            w367 = T23 0 items=["PercentOutput"=0, "Position"=1, "Velocity"=2, "Current"=3, "Follower"=5, "MotionProfile"=6, "MotionMagic"=7, "MotionMagicArc"=8, "MotionProfileArc"=10, "Disabled"=15] ("Control Mode")
            w370 = T23 0 items=["PercentOutput"=0, "Position"=1, "Velocity"=2, "Current"=3, "Follower"=5, "MotionProfile"=6, "MotionMagic"=7, "MotionMagicArc"=8, "MotionProfileArc"=10, "Disabled"=15] ("Control Mode")
            n153 = call "CTRE_Phoenix_MotorControl_Set.vi"("Output"=w366, "Control Mode"=w370, "PhoenixMotorControlDevRef"=w368) -> ()  [unwired: 7 in, 2 out]
            n154 = call "CTRE_Phoenix_MotorControl_Set.vi"("Output"=w366, "Control Mode"=w367, "PhoenixMotorControlDevRef"=w369) -> ()  [unwired: 7 in, 2 out]
          }
          frame condition #1 {
          }
          frame condition #2 {
            w373 = T23 0 items=["PercentOutput"=0, "Position"=1, "Velocity"=2, "Current"=3, "Follower"=5, "MotionProfile"=6, "MotionMagic"=7, "MotionMagicArc"=8, "MotionProfileArc"=10, "Disabled"=15] ("Control Mode")
            w375 = T23 0 items=["PercentOutput"=0, "Position"=1, "Velocity"=2, "Current"=3, "Follower"=5, "MotionProfile"=6, "MotionMagic"=7, "MotionMagicArc"=8, "MotionProfileArc"=10, "Disabled"=15] ("Control Mode")
            n155 = call "CTRE_Phoenix_MotorControl_Set.vi"("Output"=w371, "Control Mode"=w375, "PhoenixMotorControlDevRef"=w374) -> ()  [unwired: 7 in, 2 out]
            n156 = call "CTRE_Phoenix_MotorControl_Set.vi"("Output"=w371, "Control Mode"=w373, "PhoenixMotorControlDevRef"=w372) -> ()  [unwired: 7 in, 2 out]
          }
        }
      }
      frame "TowerClimbImmediate" {
        w379 = 100.0  # Wait ms
        # "Immediate command\ndoesn't need to loop.\nIf it doesn't get another\nCmd within 100ms, abort."
        n157 = Unbundle(w382) -> ("Start Time (ms)"=w385:u32)  [unwired: 1 out]
        n158 = Subtract(x=w381, y=w385) -> (x-y=w384:u32)
        n159 = Greater?(x=w384, y=u8 50 ("Left Motor")) -> (0:w380:bool)
        n160 = disable-structure shown="robot_simulation==off" {
          disable-tunnel: w377 -> [w390 _ w397]
          disable-tunnel: w378 -> [w389 _ w395]
          disable-tunnel: w376 -> [w386 _ w392]
          frame condition #0 (active) {
            w388 = T23 0 items=["PercentOutput"=0, "Position"=1, "Velocity"=2, "Current"=3, "Follower"=5, "MotionProfile"=6, "MotionMagic"=7, "MotionMagicArc"=8, "MotionProfileArc"=10, "Disabled"=15] ("Control Mode")
            w391 = T23 0 items=["PercentOutput"=0, "Position"=1, "Velocity"=2, "Current"=3, "Follower"=5, "MotionProfile"=6, "MotionMagic"=7, "MotionMagicArc"=8, "MotionProfileArc"=10, "Disabled"=15] ("Control Mode")
            # "ClimgImmediate will ONLY move winch"
            n161 = call "CTRE_Phoenix_MotorControl_Set.vi"("Output"=w389, "Control Mode"=w391, "PhoenixMotorControlDevRef"=w390) -> ()  [unwired: 7 in, 2 out]
            n162 = call "CTRE_Phoenix_MotorControl_Set.vi"("Output"=0.0, "Control Mode"=w388, "PhoenixMotorControlDevRef"=w386) -> ()  [unwired: 7 in, 2 out]
          }
          frame condition #1 {
          }
          frame condition #2 {
            w394 = T23 0 items=["PercentOutput"=0, "Position"=1, "Velocity"=2, "Current"=3, "Follower"=5, "MotionProfile"=6, "MotionMagic"=7, "MotionMagicArc"=8, "MotionProfileArc"=10, "Disabled"=15] ("Control Mode")
            w396 = T23 0 items=["PercentOutput"=0, "Position"=1, "Velocity"=2, "Current"=3, "Follower"=5, "MotionProfile"=6, "MotionMagic"=7, "MotionMagicArc"=8, "MotionProfileArc"=10, "Disabled"=15] ("Control Mode")
            n163 = call "CTRE_Phoenix_MotorControl_Set.vi"("Output"=w395, "Control Mode"=w396, "PhoenixMotorControlDevRef"=w397) -> ()  [unwired: 7 in, 2 out]
            n164 = call "CTRE_Phoenix_MotorControl_Set.vi"("Output"=0.0, "Control Mode"=w394, "PhoenixMotorControlDevRef"=w392) -> ()  [unwired: 7 in, 2 out]
          }
        }
      }
    }
    n165 = call "tower Check for New Command.vi"("Current Command"=w77, "Wait time (ms)"=w69, "Finished?"=w70) -> ("Completion"=w78:T1, "Subsystem Name"=w79:string, "Current Command"=w80:T2, "Initial Trace String"=w81:string, "NextCommand"=w82:T22)  [unwired: 4 in]
    n166 = disable-structure shown="Disabled" {
      frame Disabled {
        # "Publish"
        n167 = call-poly <vilib>:"NT Write Value.vi"() -> ()  [unwired: 11 in, 1 out]
      }
      frame Enabled {
      }
    }
    n168 = case shown="\"Successful\", \"Aborted\"" w78 {
      selector: w78 -> [_ w110]
      tunnel: w81 -> [_ w106]
      tunnel: w80 -> [_ w107]
      tunnel: w79 -> [_ w103]
      frame "Incomplete", Default {
        # "Continuing current command"
      }
      frame "Successful", "Aborted" {
        # "Report and setup for next command"
        n169 = Unbundle By Name(w107) -> ("Setpoint"=w109:dbl, "Duration"=w104:dbl)
        n170 = Format Into String(format string="S %.1f, D %f", initial string=w106, w109, w104) -> (resulting string=w105:string)  [unwired: 1 in, 1 out]
        "Current\nCmd" <- w105
        n171 = call <vilib>:"Trace Results.vi"("Status of previous command"=w110, "Description"=w105, "Subsystem"=w103) -> ()  [unwired: 9 in]
      }
    }
  }
  n172 = while {
    tunnel: w6 -> [w405]
    stop <- FALSE stop-if-true
    n173 = call "tower Controller Interactive Check.vi"("Interactive Command in"="Interactive Values", "Default Command"=w405, "Buttons"="Buttons") -> ("Interactive Command out"=w402:T2, "Trace String"=w403:string, "Schedule"=w404:bool)  [unwired: 6 in]
    n174 = case shown="True" w404 {
      tunnel: [w416 w421] -> w401
      tunnel: w402 -> [_ w419]
      tunnel: [w412 w417] -> w400
      tunnel: w403 -> [_ w420]
      frame False {
        n175 = Tick Count (ms)() -> (millisecond timer value=w411:u32)
        n176 = call "Read tower Operation.vi"() -> ("Command Info"=w410:T20, "Command Timing"=w409:cluster{"Start Time (ms)":u32, "Iterations":i32})  [unwired: 9 in, 1 out]
        n177 = Unbundle(w409) -> ("Start Time (ms)"=w415:u32, "Iterations"=w413:i32)
        n178 = Unbundle(w410) -> ("Status"=w416:T1)  [unwired: 2 out]
        n179 = Subtract(x=w411, y=w415) -> (x-y=w414:u32)
        n180 = Bundle(w414, "Iterations"=w413) -> (w412:cluster{u32, "Iterations":i32})  [unwired: 1 in]
      }
      frame True {
        n181 = call "tower Command Helper.vi"("Description"=w420, "SubSystem Data"=w419) -> ("Command Info Out"=w418:T20, "Command Timing"=w417:cluster{"Start Time (ms)":u32, "Iterations":i32})  [unwired: 7 in, 1 out]
        n182 = Unbundle(w418) -> ("Status"=w421:T1)  [unwired: 2 out]
      }
    }
    "Status" <- w401
    "Command Timing" <- w400
    n183 = global read "tower Published Globals.vi" "TowerLastCommandStatus"() -> (→"TowerLastCommandStatus":T1)
    n184 = Wait (ms)(milliseconds to wait=u32 20) -> ()  [unwired: 1 out]
  }
